vi "Get Metrics.vi"(7 "LabVIEW Web Service Request":refnum<class "Web Request.lvclass">, 11 "Registry":string="_default_registry") -> ()   [LabVIEW 2020]
uses:
  <vilib>/wsapi/Web Request.lvclass
  <vilib>/Utility/error.llb/DialogType.ctl
  <vilib>/TheLabVIEWLab/PromVIEW/registry/session/Registry Session.lvclass
  <vilib>/TheLabVIEWLab/PromVIEW/metrics/metric/Metric.lvclass
panel:
  # "Use the Web Service Request input terminal to call the VIs on the Web Services palette. Do not remove it from the connector pane unless you don't need access to the palette."
  # "Each additional control wired to the connector pane will be available as an input in the URL. To include an indicator in terminal-mode output (the default setting), it must also be wired to the connector pane."
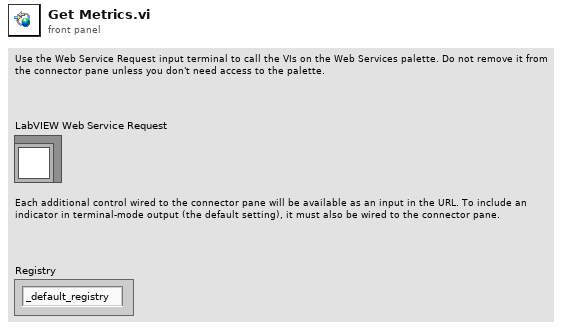
[diagram p1: front panel]
types:
  T1 = typedef "Registry.lvlib/Registry Session.lvclass/Session Handle.ctl" = refnum<data-value>
  T2 = typedef "DialogType.ctl" = u16
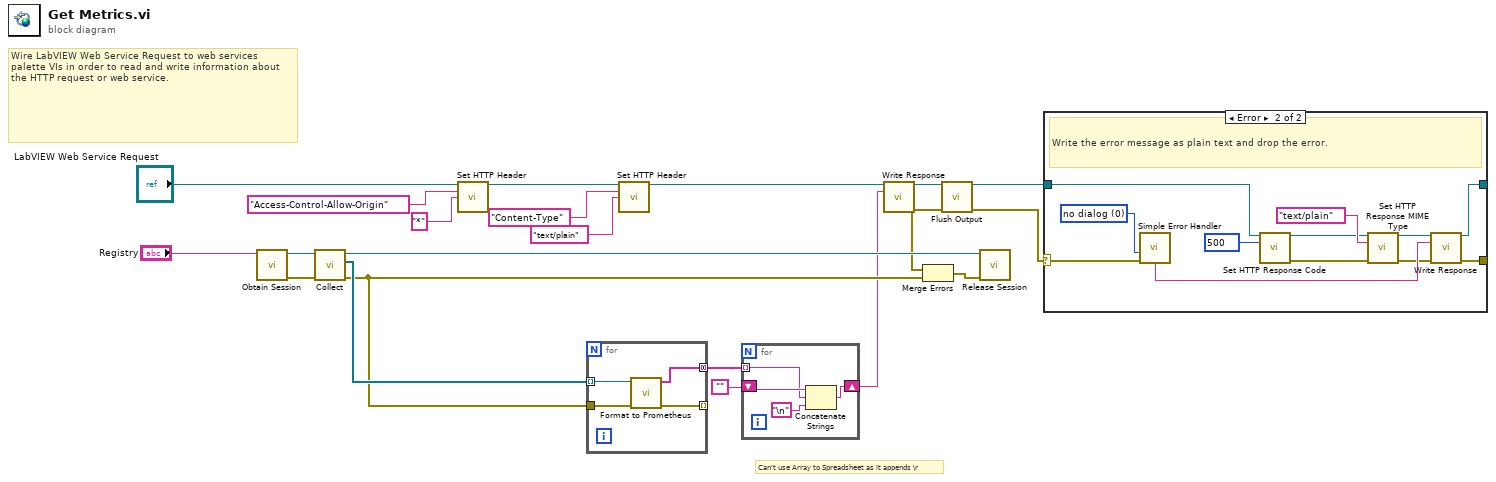
[diagram p0: block diagram]
diagram:
  # "Can't use Array to Spreadsheet as it appends \\r"
  # "Wire LabVIEW Web Service Request to web services palette VIs in order to read and write information about the HTTP request or web service."
  n1 = call <vilib>:"Obtain Session.vi"("Session  Name ()"="Registry") -> ("error out"=w16:errorcluster, "Session Handle"=w17:T1)  [unwired: 9 in]
  n2 = call <vilib>:"Collect.vi"("error in (no error)"=w16, "Session Handle in"=w17) -> ("error out"=w6:errorcluster, "Metrics"=w15:refnum<data-value>[], "Session Handle out"=w14:T1)  [unwired: 7 in]
  n3 = call <vilib>:"Set HTTP Header.vi"("LabVIEW Web Service Request"="LabVIEW Web Service Request", "header"="Access-Control-Allow-Origin", "header value"="*") -> ("LabVIEW Web Service Request out"=w10:refnum<class "Web Request.lvclass">)  [unwired: 11 in, 1 out]
  n4 = for {
    tunnel: w15 -> [w25] mode=indexing
    tunnel: [w24] -> w3 mode=concatenating
    tunnel: w6 -> [w23]
    tunnel: [w22] -> _ mode=indexing
    n5 = call <vilib>:"Format to Prometheus.vi"("error in (no error)"=w23, "Metric"=w25) -> ("error out"=w22:errorcluster, "Prometheus-formatted Metric"=w24:string[])  [unwired: 8 in]
  }
  n6 = call <vilib>:"Set HTTP Header.vi"("LabVIEW Web Service Request"=w10, "header"="Content-Type", "header value"="text/plain") -> ("LabVIEW Web Service Request out"=w9:refnum<class "Web Request.lvclass">)  [unwired: 11 in, 1 out]
  n7 = for {
    tunnel: w3 -> [w27] mode=indexing
    shift-right: [w26] -> w4
    shift-left: "" -> [w29]
    n8 = Concatenate Strings(w29, w27, "\n") -> (w26:string)
  }
  n9 = call <vilib>:"Write Response.vi"("LabVIEW Web Service Request"=w9, "response string"=w4) -> ("LabVIEW Web Service Request out"=w13:refnum<class "Web Request.lvclass">, "error out"=w7:errorcluster)  [unwired: 12 in]
  n10 = Merge Errors(w7, w6) -> (w8:errorcluster)
  n11 = call <vilib>:"Flush Output.vi"("LabVIEW Web Service Request"=w13, "error in (no error)"=w7) -> ("LabVIEW Web Service Request out"=w2:refnum<class "Web Request.lvclass">, "error out"=w1:errorcluster)  [unwired: 12 in]
  n12 = call <vilib>:"Release Session.vi"("error in (no error)"=w8, "Session Handle"=w14) -> ()  [unwired: 9 in, 1 out]
  n13 = case shown="Error" w1 {
    selector: w1 -> [w30 w39]
    tunnel: w2 -> [w31 w34]
    tunnel: [w31 w41] -> _
    tunnel: [w30 w40] -> _
    frame No Error {
      # "Nothing to do when there is no error."
    }
    frame Error {
      w35 = 500 items=["100"=100, "101"=101, "200"=200, "201"=201, "202"=202, "203"=203, "204"=204, "205"=205, "206"=206, "300"=300, "301"=301, "302"=302, "303"=303, "304"=304, "305"=305, "306"=306, "307"=307, "400"=400, "401"=401, "402"=402, "403"=403, "404"=404, "405"=405, "406"=406, "407"=407, "408"=408, "409"=409, "410"=410, "411"=411, "412"=412, "413"=413, "414"=414, "415"=415, "416"=416, "417"=417, "500"=500, "501"=501, "502"=502, "503"=503, "504"=504, "505"=505] ("response code (200)")
      w42 = T2 0 items=["no dialog", "OK message", "continue or stop message", "OK message + warnings", "continue/stop + warnings"] ("type of dialog (OK msg:1)")
      # "Write the error message as plain text and drop the error."
      n14 = call <vilib>:"Simple Error Handler.vi"("type of dialog (OK msg:1)"=w42, "error in (no error)"=w39) -> ("message"=w43:string)  [unwired: 3 in, 4 out]
      n15 = call <vilib>:"Set HTTP Response Code.vi"("LabVIEW Web Service Request"=w34, "response code (200)"=w35) -> ("LabVIEW Web Service Request out"=w33:refnum<class "Web Request.lvclass">, "error out"=w36:errorcluster)  [unwired: 12 in]
      n16 = call <vilib>:"Set HTTP Response MIME Type.vi"("LabVIEW Web Service Request"=w33, "MIME type (text/html)"="text/plain", "error in (no error)"=w36) -> ("LabVIEW Web Service Request out"=w32:refnum<class "Web Request.lvclass">, "error out"=w38:errorcluster)  [unwired: 11 in]
      n17 = call <vilib>:"Write Response.vi"("LabVIEW Web Service Request"=w32, "response string"=w43, "error in (no error)"=w38) -> ("LabVIEW Web Service Request out"=w41:refnum<class "Web Request.lvclass">, "error out"=w40:errorcluster)  [unwired: 11 in]
    }
  }
